vi "calibrate_on_command.vi"() -> (0 "error out":errorcluster)   [LabVIEW 2013]
panel:
  out "Image":T1(plugin-control)
  in  "Calibrate":bool
  in  "File Path (Image Calibration 1)":path=path "\\\\hs2.lboro.ac.uk\\mmbc4/1_Univesity Work/Mechatronics/Machine Vision/Harry_Kane_Project/A3_table_cal_2.png"
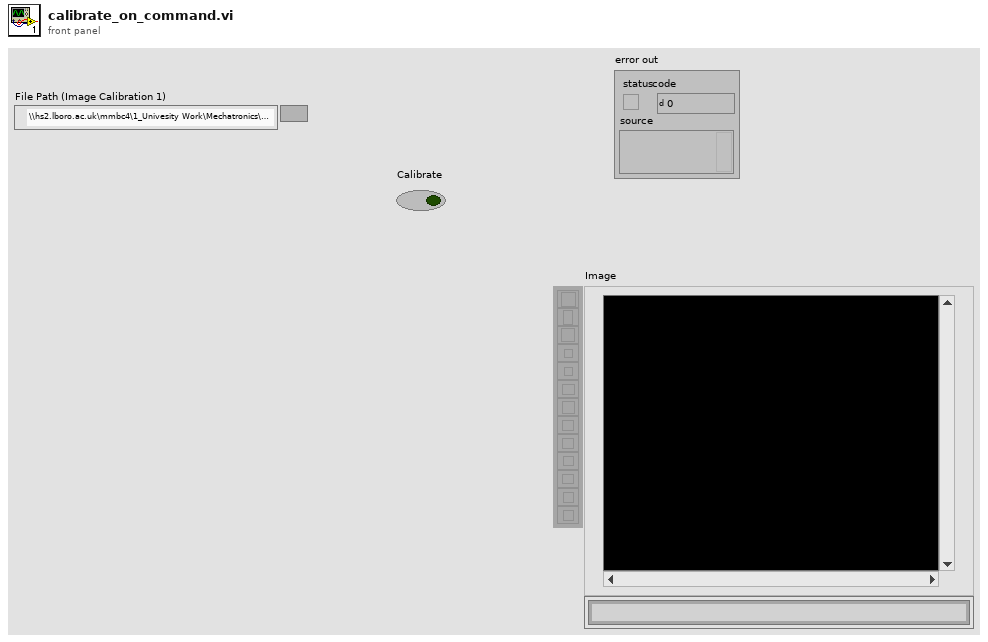
[diagram p1: front panel]
types:
  T1 = typedef "IMAQ Image.ctl" = refnum<image>
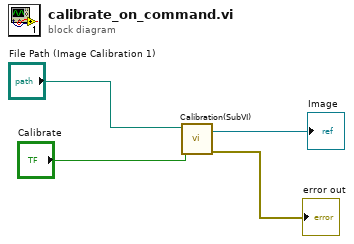
[diagram p0: block diagram]
diagram:
  n1 = call "Calibration(SubVI).vi"("Calibrate"="Calibrate", "File Path (Image Calibration 1)"="File Path (Image Calibration 1)") -> ("error out"=→"error out":errorcluster, "Refnum out"=→"Image":T1)  [unwired: 8 in]
